vi "get configuration by UID.vi"(8 "error in":errorcluster, 10 "UID":string, 11 "NISE_CEF_HierarchyRepo in":refnum<class "NISE_CEF_HierarchyRepo.lvclass">) -> (0 "error out":errorcluster, 1 "configuration":refnum<class "NISE_CEF_serializable configuration.lvclass">, 3 "NISE_CEF_HierarchyRepo out":refnum<class "NISE_CEF_HierarchyRepo.lvclass">)   [LabVIEW 2013, in "NISE_CEF_HierarchyRepo.lvclass"]
uses:
  NISE_CEF_HierarchyRepo.lvclass
  serializable configuration/NISE_CEF_serializable configuration.lvclass
  NISE_CEF_HierarchyRepo.lvclass/NISE_CEF_HierarchyRepo.ctl
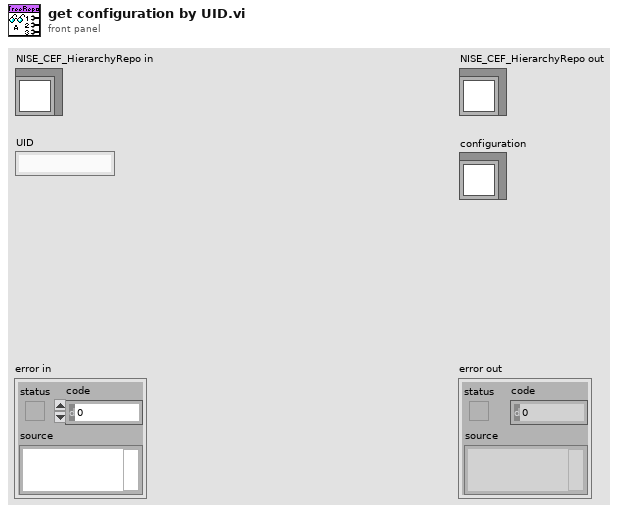
[diagram p1: front panel]
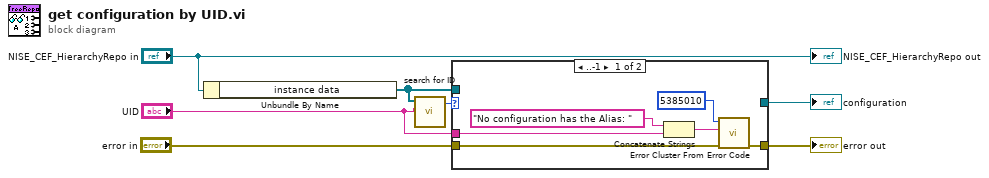
[diagram p0: block diagram]
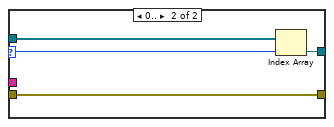
[diagram p2: hidden frame]
diagram:
  n1 = Unbundle By Name("NISE_CEF_HierarchyRepo in") -> ("instance data"=w1:refnum<class "NISE_CEF_serializable configuration.lvclass">[])
  n2 = call "search for ID.vi"("instance id"="UID", "instance data"=w1) -> ("index"=w2:i32)  [unwired: 9 in]
  n3 = case shown="..-1" w2 {
    selector: w2 -> [_ w14]
    tunnel: w1 -> [_ w17]
    tunnel: [_ w16] -> w3
    tunnel: "error in" -> [w13 w15]
    tunnel: [w12 w15] -> w6
    tunnel: "UID" -> [w9 _]
    frame ..-1 {
      n4 = Concatenate Strings("No configuration has the Alias: " ("string"), w9) -> (w10:string)
      n5 = call <vilib>:"Error Cluster From Error Code.vi"("error in (no error)"=w13, "error message (\"\")"=w10, "error code (0)"=5385010) -> ("error out"=w12:errorcluster)  [unwired: 6 in]
    }
    frame 0.. {
      n6 = Index Array(array=w17, index=w14) -> (element=w16:refnum<class "NISE_CEF_serializable configuration.lvclass">)
    }
  }
  "error out" <- w6
  "configuration" <- w3
  "NISE_CEF_HierarchyRepo out" <- "NISE_CEF_HierarchyRepo in"
